vi "Main_07b.vi"() -> ()   [LabVIEW 2020]
uses:
  file_Item/MAP_Structure.ctl
  file_Item/Cluster_Item Data.ctl
  582f8871-3865-485f-b414-23c64cb36c00.vi
  acaf9b7b-e7cc-406a-a77a-e34bba61f78d.vi
  <vilib>/Comparison/Less/Less Functor/Less Functor.lvclass
  <vilib>/Comparison/Equal/Equal Functor/Equal Functor.lvclass
panel:
  out "index of element":i32
  out "\\ Size":u32
  out "sorted array":u32[](array[numeric])
  out "Selected dir size":u32
  out "target number for unused":u32
  out "Free Space":u32
  out "Map":T1
  out "array":string[](array[string])
  in  "Puzzle":string="$ cd /\n$ ls\n187585 dgflmqwt.srm\ndir gnpd\n200058 hbnlqs\ndir jsv\ndir mfhzl\ndir nljtr\ndir nwzp\n61949 qdswp.wfj\n21980 rbq.hpj\ndir rfwwwgr\ndir sbnhc\ndir zhfl\n136762 zwg\n$ cd gnpd\n$ ls\ndir dcqq\ndir dnscfz\ndir dwqbhgc\ndir lsrb\n167581 ndwfr.pbv\ndir pbgrdvmc\ndir sbnhc\n144703 sct\ndir smfhldss\n$ cd dcqq\n$ ls\ndir bfdng\n155230 mfhzl.bpw\ndir mhpqqq\ndir mpbpcv\n24140 mrrznmvr.mmz\n$ cd bfdng\n$ ls\ndir hjlch\ndir sbnhc\n$ cd hjlch\n$ ls\n239759 sct\n$ cd ..\n$ cd sbnhc\n$ ls\n221334 hbnlqs\n$ cd ..\n$ cd ..\n$ cd mhpqqq\n$ ls\n250305 nfqs.crt\ndir qqhz\n60892 rbq.hpj\n64587 tbzlnq\ndir tcbgmw\ndir vnlmlq\n$ cd qqhz\n$ ls\n148009 sct\n$ cd ..\n$ cd tcbgmw\n$ ls\n85006 sbnhc\n$ cd ..\n$ cd vnlmlq\n$ ls\n21720 vsrrhvlt.qbs\n$ cd ..\n$ cd ..\n$ cd mpbpcv\n$ ls\n146794 bdpld.ddm\n$ cd ..\n$ cd ..\n$ cd dnscfz\n$ ls\n276175 mfhzl.ndh\n248161 qjgzgm\ndir vnlmlq\ndir wwf\ndir zjdhldlq\n$ cd vnlmlq\n$ ls\n130051 ftjnfc\n$ cd ..\n$ cd wwf\n$ ls\n166550 dwvphbm.jtd\n$ cd ..\n$ cd zjdhldlq\n$ ls\n345090 hbnlqs\n$ cd ..\n$ cd ..\n$ cd dwqbhgc\n$ ls\n310228 dwvphbm\n157686 hbnlqs\n48014 nfqs.crt\n333356 rwb.njl\ndir sbnhc\n139174 sct\ndir vjcl\n$ cd sbnhc\n$ ls\n51605 bfqw.cjd\n267184 fjvmbpf\n169122 mfhzl.jrp\n243630 sbnhc\n$ cd ..\n$ cd vjcl\n$ ls\ndir mfhzl\n$ cd mfhzl\n$ ls\n302243 dcqq.djc\n$ cd ..\n$ cd ..\n$ cd ..\n$ cd lsrb\n$ ls\n311814 dcqq.prd\n200118 rbq.hpj\n$ cd ..\n$ cd pbgrdvmc\n$ ls\n119324 cqhdvmzp.npw\n277930 jhlrpmqg\ndir jlcqmq\n204425 pddmq\ndir rqmhwhc\n257084 sbnhc\n338348 vnlmlq\n$ cd jlcqmq\n$ ls\n24876 mfhzl\n$ cd ..\n$ cd rqmhwhc\n$ ls\n36575 dlft.dtp\n$ cd ..\n$ cd ..\n$ cd sbnhc\n$ ls\ndir sbq\ndir vmslnrmc\n$ cd sbq\n$ ls\n15689 hpzgsl.svb\n$ cd ..\n$ cd vmslnrmc\n$ ls\ndir lcqpws\n136481 nfqs.crt\n29838 sbnhc\n$ cd lcqpws\n$ ls\n168866 dcqq.pdp\n322264 jmtwr.fzj\n18732 sct\n$ cd ..\n$ cd ..\n$ cd ..\n$ cd smfhldss\n$ ls\ndir wfbssqj\n$ cd wfbssqj\n$ ls\n134050 tgghrp.hjq\n$ cd ..\n$ cd ..\n$ cd ..\n$ cd jsv\n$ ls\ndir bwc\ndir dcqq\n260913 lzcqm.wzr\ndir rhstw\ndir vnlmlq\n$ cd bwc\n$ ls\n221975 bdv.mfq\ndir crbnzrtw\ndir dcqq\ndir gdgh\n101246 gqcfrzmn\ndir gsst\ndir jwrhclh\ndir nbwfdvsv\ndir qnwhfv\ndir sbnhc\n$ cd crbnzrtw\n$ ls\ndir dmmpcrz\n204859 dwvphbm.csz\ndir jdh\ndir mpgdhg\n202360 nfqs.crt\ndir sbnhc\n302165 scpq.gpd\ndir shfhmdw\ndir wmjgmd\n$ cd dmmpcrz\n$ ls\ndir mfhzl\n$ cd mfhzl\n$ ls\n121861 hbnlqs\n$ cd ..\n$ cd ..\n$ cd jdh\n$ ls\ndir dwvphbm\n$ cd dwvphbm\n$ ls\n8977 ntdtdq\n$ cd ..\n$ cd ..\n$ cd mpgdhg\n$ ls\n48235 dcqq\n$ cd ..\n$ cd sbnhc\n$ ls\ndir dbb\n$ cd dbb\n$ ls\n275648 gcsdd.pdw\ndir rbbgrtm\ndir rmlm\n111336 sbnhc.qrn\n153146 sct\n$ cd rbbgrtm\n$ ls\n304685 rbq.hpj\n$ cd ..\n$ cd rmlm\n$ ls\ndir wfr\n$ cd wfr\n$ ls\n197220 dhjjr.dqq\n$ cd ..\n$ cd ..\n$ cd ..\n$ cd ..\n$ cd shfhmdw\n$ ls\n221308 mhnfzmz.gqp\n$ cd ..\n$ cd wmjgmd\n$ ls\ndir psrshrws\ndir zrtpgbg\n$ cd psrshrws\n$ ls\n202052 twgfblm\n$ cd ..\n$ cd zrtpgbg\n$ ls\n48134 hsnzvhvm.gnp\n$ cd ..\n$ cd ..\n$ cd ..\n$ cd dcqq\n$ ls\n63600 tlclsj.pvg\n181384 tzjn\n90096 wgq.lrm\n$ cd ..\n$ cd gdgh\n$ ls\n78450 hrcdgnpv.ctz\n$ cd ..\n$ cd gsst\n$ ls\n345240 nfqs.crt\n199259 sct\n$ cd ..\n$ cd jwrhclh\n$ ls\ndir ftjcr\n177499 nhdh.bbn\ndir sbnhc\ndir vnlmlq\ndir wqjnwgpj\n$ cd ftjcr\n$ ls\ndir glfptjpb\n121761 gqp\n36602 lcgfmtf.zct\ndir mfhzl\ndir rrrrgbqv\n236133 wdmwgzvs.jnw\ndir zwrmjlh\n$ cd glfptjpb\n$ ls\ndir fdnppcr\ndir gchhnd\ndir gdphvds\n98000 gqhv\n$ cd fdnppcr\n$ ls\ndir dwvphbm\ndir ngsgrgp\n$ cd dwvphbm\n$ ls\ndir wrg\n$ cd wrg\n$ ls\n265022 cqhdvmzp.npw\n316916 nfqs.crt\n$ cd ..\n$ cd ..\n$ cd ngsgrgp\n$ ls\n110198 sct\n$ cd ..\n$ cd ..\n$ cd gchhnd\n$ ls\n253836 hbnlqs\n39462 mfhzl\n211458 nfqs.crt\n$ cd ..\n$ cd gdphvds\n$ ls\ndir dpdb\n$ cd dpdb\n$ ls\n342610 vnlmlq\n$ cd ..\n$ cd ..\n$ cd ..\n$ cd mfhzl\n$ ls\ndir cptj\n$ cd cptj\n$ ls\n100729 nvctqj.gjw\n$ cd ..\n$ cd ..\n$ cd rrrrgbqv\n$ ls\n166055 dwvphbm.rvb\n303762 hbnlqs\n277411 wzr.rgz\n$ cd ..\n$ cd zwrmjlh\n$ ls\n32583 dvfnw\n$ cd ..\n$ cd ..\n$ cd sbnhc\n$ ls\ndir hwtmwp\n334229 mfhzl\n299303 vtrfbw.dng\n$ cd hwtmwp\n$ ls\ndir zjmrr\n$ cd zjmrr\n$ ls\n279103 cqhdvmzp.npw\n$ cd ..\n$ cd ..\n$ cd ..\n$ cd vnlmlq\n$ ls\ndir btqsh\ndir clhclcr\n237487 cqhdvmzp.npw\n11669 gqhltqf\n91205 hbnlqs\ndir qwbnvzv\n234450 rqlnhpc.qfd\ndir vbrc\ndir vfdqq\n$ cd btqsh\n$ ls\ndir lgh\ndir ljrjpg\n34333 rbq.hpj\n15387 vzldp.ffs\n$ cd lgh\n$ ls\n176966 vnlmlq\n$ cd ..\n$ cd ljrjpg\n$ ls\n231230 cqhdvmzp.npw\ndir dwvphbm\ndir mfhzl\n251554 rdrbn.clr\n180447 sbnhc\n$ cd dwvphbm\n$ ls\ndir vghvsmq\n$ cd vghvsmq\n$ ls\n132209 cqhdvmzp.npw\ndir jqmgn\n$ cd jqmgn\n$ ls\n95992 clbvg.bmr\n$ cd ..\n$ cd ..\n$ cd ..\n$ cd mfhzl\n$ ls\ndir dcqq\n$ cd dcqq\n$ ls\ndir vjhl\n$ cd vjhl\n$ ls\ndir nbhmzl\n$ cd nbhmzl\n$ ls\n155454 sbnhc.flh\n$ cd ..\n$ cd ..\n$ cd ..\n$ cd ..\n$ cd ..\n$ cd ..\n$ cd clhclcr\n$ ls\ndir jwqwhq\n268077 njcmcfl.ctm\n$ cd jwqwhq\n$ ls\n256988 rbq.hpj\n$ cd ..\n$ cd ..\n$ cd qwbnvzv\n$ ls\n167852 dln.zrn\ndir hpwpm\n131149 lsc.tjj\ndir mfhzl\ndir mzhwwrtp\n201277 sbnhc.pfh\n147232 zlmgttpl\n$ cd hpwpm\n$ ls\n135194 jpzt.fjn\n$ cd ..\n$ cd mfhzl\n$ ls\n166015 jrcqvgf.jdg\n$ cd ..\n$ cd mzhwwrtp\n$ ls\n231983 dgrvfdmp\n121846 dwvphbm.lvp\n$ cd ..\n$ cd ..\n$ cd vbrc\n$ ls\n320029 wbhs.mpd\n$ cd ..\n$ cd vfdqq\n$ ls\n277998 nfqs.crt\ndir qzgwglhc\ndir vnlmlq\n68520 wsc.vhz\ndir zfdhthfn\n$ cd qzgwglhc\n$ ls\n25046 cqhdvmzp.npw\n250876 dwvphbm\n$ cd ..\n$ cd vnlmlq\n$ ls\n212688 hbnlqs\n8202 mlpl.tsp\n69495 vnlmlq.thv\n281200 vzdwr.tbl\n$ cd ..\n$ cd zfdhthfn\n$ ls\n233242 dstb.hrs\n269387 nfqs.crt\n$ cd ..\n$ cd ..\n$ cd ..\n$ cd wqjnwgpj\n$ ls\ndir hfd\ndir lbft\ndir rtlw\ndir vbf\n$ cd hfd\n$ ls\n224694 cqhdvmzp.npw\n100103 dbmwn.tqz\n$ cd ..\n$ cd lbft\n$ ls\n60107 hbnlqs\n$ cd ..\n$ cd rtlw\n$ ls\ndir ntpb\n$ cd ntpb\n$ ls\n341166 mfhzl.pvj\n$ cd ..\n$ cd ..\n$ cd vbf\n$ ls\n54177 ghrscj.tlh\n$ cd ..\n$ cd ..\n$ cd ..\n$ cd nbwfdvsv\n$ ls\n107273 mptw.qmn\n$ cd ..\n$ cd qnwhfv\n$ ls\n55633 hbnlqs\n$ cd ..\n$ cd sbnhc\n$ ls\n173163 vnlmlq\n$ cd ..\n$ cd ..\n$ cd dcqq\n$ ls\n217679 hbnlqs\n146747 ltp\n$ cd ..\n$ cd rhstw\n$ ls\ndir clh\ndir grz\ndir ntjtzr\ndir qrjgl\ndir rzqp\ndir tzgrs\ndir zrdh\n$ cd clh\n$ ls\n212153 cqhdvmzp.npw\n$ cd ..\n$ cd grz\n$ ls\n346002 cqhdvmzp.npw\n$ cd ..\n$ cd ntjtzr\n$ ls\n271549 rbq.hpj\n308693 sbnhc.zrv\n$ cd ..\n$ cd qrjgl\n$ ls\n119344 jfshwj\n$ cd ..\n$ cd rzqp\n$ ls\n327891 dcqq\n210282 hlmnv.jph\n118199 nfqs.crt\ndir rwh\n$ cd rwh\n$ ls\n285057 rmvrnb\n$ cd ..\n$ cd ..\n$ cd tzgrs\n$ ls\n23830 cjqrr\n$ cd ..\n$ cd zrdh\n$ ls\ndir dcqq\ndir dwvphbm\n188911 rbq.hpj\ndir vpnzs\n$ cd dcqq\n$ ls\n277454 hbnlqs\ndir jnncgzgm\n$ cd jnncgzgm\n$ ls\n199664 dcqq.tgm\n$ cd ..\n$ cd ..\n$ cd dwvphbm\n$ ls\n221700 fgnznr.dhf\n$ cd ..\n$ cd vpnzs\n$ ls\n254459 fvcf.zcj\n$ cd ..\n$ cd ..\n$ cd ..\n$ cd vnlmlq\n$ ls\ndir gfsj\n$ cd gfsj\n$ ls\ndir hddvr\n$ cd hddvr\n$ ls\ndir mqmnzb\n$ cd mqmnzb\n$ ls\n341835 jjjh\n$ cd ..\n$ cd ..\n$ cd ..\n$ cd ..\n$ cd ..\n$ cd mfhzl\n$ ls\ndir pccldwf\n$ cd pccldwf\n$ ls\n126977 nvcw\n318605 rljpfnc.dzd\n$ cd ..\n$ cd ..\n$ cd nljtr\n$ ls\ndir slztzqd\n$ cd slztzqd\n$ ls\n55754 bpwghjpg.bfq\n205753 pfplh\n319151 vdlmjj.mmn\ndir vnlmlq\n$ cd vnlmlq\n$ ls\ndir mfhzl\n338081 zhjrrs\ndir zpj\n$ cd mfhzl\n$ ls\ndir dcqq\ndir lgfb\ndir rjbprpnl\n343125 vnlmlq.zpr\n$ cd dcqq\n$ ls\n288030 rbq.hpj\n$ cd ..\n$ cd lgfb\n$ ls\n22119 cqhdvmzp.npw\n238775 wbmnzgt.vnl\n$ cd ..\n$ cd rjbprpnl\n$ ls\n244896 lvgg.jvz\n$ cd ..\n$ cd ..\n$ cd zpj\n$ ls\n339679 dcqq\n$ cd ..\n$ cd ..\n$ cd ..\n$ cd ..\n$ cd nwzp\n$ ls\ndir mfhzl\ndir vnlmlq\n$ cd mfhzl\n$ ls\n107297 dwvphbm.nvb\n$ cd ..\n$ cd vnlmlq\n$ ls\ndir mdj\n$ cd mdj\n$ ls\n87553 dbtct.nws\n$ cd ..\n$ cd ..\n$ cd ..\n$ cd rfwwwgr\n$ ls\n287719 flpwrp\n74896 mfhzl\n$ cd ..\n$ cd sbnhc\n$ ls\n232949 dcqq.rnj\ndir dwvphbm\n$ cd dwvphbm\n$ ls\n21955 pcqbfbv.bfg\n$ cd ..\n$ cd ..\n$ cd zhfl\n$ ls\ndir jvnlhq\ndir vnlmlq\n180619 wcd.jsr\n$ cd jvnlhq\n$ ls\n20692 clp.vmd\ndir dbn\n91389 jqbp.zss\ndir njmdrb\ndir sbnhc\ndir sdrrzp\n192374 vnlmlq.lvj\n$ cd dbn\n$ ls\n293401 dcqq\n$ cd ..\n$ cd njmdrb\n$ ls\n270463 dvzbtnbb.vth\ndir gdvtg\n219739 hsdg.rss\ndir mfhzl\n285584 mhq\ndir mllvdccz\n234503 nfqs.crt\n$ cd gdvtg\n$ ls\n294243 dllnh\n27407 rws.vqt\n$ cd ..\n$ cd mfhzl\n$ ls\ndir dwvphbm\n154477 nbphv.pjc\ndir qpnncj\n33994 splscqn.tqz\ndir vnlmlq\n$ cd dwvphbm\n$ ls\n87960 sct\n$ cd ..\n$ cd qpnncj\n$ ls\n182692 lqbbz\n$ cd ..\n$ cd vnlmlq\n$ ls\n285614 bfrjhpv.dvn\n121146 nfqs.crt\n84544 sbnhc\n$ cd ..\n$ cd ..\n$ cd mllvdccz\n$ ls\n184878 bsjzsmw.pwt\n184061 dcqq.bbm\n243546 dwvphbm.rdw\ndir ftmrszgl\n8251 rbq.hpj\ndir tgvchzn\n$ cd ftmrszgl\n$ ls\n267439 bdrn.gfb\n257447 npcrg.gjn\n$ cd ..\n$ cd tgvchzn\n$ ls\n227775 lqbftlg.scr\n$ cd ..\n$ cd ..\n$ cd ..\n$ cd sbnhc\n$ ls\n245520 tjp.pml\n$ cd ..\n$ cd sdrrzp\n$ ls\ndir dcqq\n7894 gstzs\ndir rnjcrjj\ndir sbnhc\n$ cd dcqq\n$ ls\n340987 sjb.nss\n$ cd ..\n$ cd rnjcrjj\n$ ls\n67782 rbq.hpj\n$ cd ..\n$ cd sbnhc\n$ ls\n156705 zwr.rtg\n$ cd ..\n$ cd ..\n$ cd ..\n$ cd vnlmlq\n$ ls\ndir dwvphbm\ndir jgc\ndir lbh\ndir lrwt\ndir rhszw\n213882 sbnhc.dzl\ndir vnlmlq\n2798 vwwbhsnb.dms\n$ cd dwvphbm\n$ ls\n257972 zccsn.bdr\n$ cd ..\n$ cd jgc\n$ ls\n85911 cqhdvmzp.npw\ndir fnvjv\n49760 grsw\ndir ntz\n249818 rgzqq.tlr\n$ cd fnvjv\n$ ls\n288935 dcqq.bsq\ndir nwlbbwtq\n264238 tcwwzs.zwg\n$ cd nwlbbwtq\n$ ls\ndir qcm\n318151 sbnhc.lwr\n322077 stb.cqj\n$ cd qcm\n$ ls\n147721 crrdn\ndir gctnt\n59476 rbq.hpj\ndir sbnhc\n$ cd gctnt\n$ ls\n328909 dwvphbm\n82536 rjnz\n$ cd ..\n$ cd sbnhc\n$ ls\n35956 nfqs.crt\n89464 qvhvlcl.nzq\ndir vvn\n$ cd vvn\n$ ls\n119247 fztlb.qch\n79030 vnlmlq\n$ cd ..\n$ cd ..\n$ cd ..\n$ cd ..\n$ cd ..\n$ cd ntz\n$ ls\n234879 mfhzl\n$ cd ..\n$ cd ..\n$ cd lbh\n$ ls\ndir dwvphbm\n24310 jgsp.ggs\ndir lft\n$ cd dwvphbm\n$ ls\n295434 rbq.hpj\n$ cd ..\n$ cd lft\n$ ls\ndir dcqq\ndir dwvphbm\n123657 mfhzl.nhq\n$ cd dcqq\n$ ls\ndir tgp\n$ cd tgp\n$ ls\n271647 gmmq.tmp\n$ cd ..\n$ cd ..\n$ cd dwvphbm\n$ ls\ndir pftcdtd\n108321 qtqhqwnt\n$ cd pftcdtd\n$ ls\n28073 hwqzcr.zcp\n$ cd ..\n$ cd ..\n$ cd ..\n$ cd ..\n$ cd lrwt\n$ ls\n38953 hzhzfw.tpv\n59885 vnlmlq\n$ cd ..\n$ cd rhszw\n$ ls\ndir hsfbh\ndir mmflqvsd\n20071 rhdbms\n162563 rpjjld\ndir vnlmlq\n$ cd hsfbh\n$ ls\n255050 lglw.jvw\n99814 pzvw\n28443 sbct.hng\n168934 sbnhc.fnt\ndir wnwztl\n$ cd wnwztl\n$ ls\ndir brwhjj\n215806 dcqq\n214967 mqhv.wwq\n82998 vcm.mhc\n$ cd brwhjj\n$ ls\n171935 rbq.hpj\n$ cd ..\n$ cd ..\n$ cd ..\n$ cd mmflqvsd\n$ ls\n109141 dcqq.mdc\n$ cd ..\n$ cd vnlmlq\n$ ls\ndir blggqt\n117656 dcqq.vlg\ndir fpw\n195879 gsb.dvw\ndir mfhzl\n5068 mnfdf\ndir mtg\ndir vnlmlq\n$ cd blggqt\n$ ls\n195700 ntv.zjn\n$ cd ..\n$ cd fpw\n$ ls\n143105 sct\n$ cd ..\n$ cd mfhzl\n$ ls\ndir cpcczt\n47767 nzzcn.qhp\ndir zdv\n$ cd cpcczt\n$ ls\n209755 vnlmlq.lbw\n$ cd ..\n$ cd zdv\n$ ls\n335546 sbnhc.ccg\n$ cd ..\n$ cd ..\n$ cd mtg\n$ ls\n244632 dcqq.frr\n240873 tpvqthc.ljw\ndir zdtnqtcw\n$ cd zdtnqtcw\n$ ls\n80980 nfqs.crt\n$ cd ..\n$ cd ..\n$ cd vnlmlq\n$ ls\n153953 dwvphbm\n$ cd ..\n$ cd ..\n$ cd ..\n$ cd vnlmlq\n$ ls\ndir dcqq\ndir dwvphbm\n155333 mmhjscr.mrh\n293720 nfqs.crt\ndir qnv\ndir rdvq\n226720 zgmtqvws\n160920 zgnft\n$ cd dcqq\n$ ls\n142227 cqhdvmzp.npw\n199798 twqppvs\n$ cd ..\n$ cd dwvphbm\n$ ls\n58807 cdbdnrqh.fgq\n224321 hbnlqs\n340073 sbnhc\n337932 sct\n2613 vdc.nwz\n$ cd ..\n$ cd qnv\n$ ls\n244311 cqhdvmzp.npw\n273687 jhqt.glz\ndir mnrh\n240044 nfqs.crt\n49861 pwsgmlq.hcw\ndir rdrs\n126195 vnlmlq.frr\n$ cd mnrh\n$ ls\n276125 hbnlqs\n$ cd ..\n$ cd rdrs\n$ ls\ndir dqgw\n213018 dwvphbm\n13785 hbnlqs\ndir lbpjczw\n116081 nfqs.crt\n154367 rbq.hpj\n77634 sct\n$ cd dqgw\n$ ls\ndir rpcfdr\n$ cd rpcfdr\n$ ls\ndir swvlhbg\n$ cd swvlhbg\n$ ls\n309244 sct\n$ cd ..\n$ cd ..\n$ cd ..\n$ cd lbpjczw\n$ ls\n69436 rbq.hpj\n$ cd ..\n$ cd ..\n$ cd ..\n$ cd rdvq\n$ ls\n128806 dcqq.qzr\n64132 dcqq.vgc\ndir hht\n165359 jzj.rqv\ndir sbnhc\n$ cd hht\n$ ls\ndir vnlmlq\n$ cd vnlmlq\n$ ls\n49895 wct\n$ cd ..\n$ cd ..\n$ cd sbnhc\n$ ls\n265434 vnlmlq"
  in  "Example":string="$ cd /\n$ ls\ndir a\n14848514 b.txt\n8504156 c.dat\ndir d\n$ cd a\n$ ls\ndir e\n29116 f\n2557 g\n62596 h.lst\n$ cd e\n$ ls\n584 i\n$ cd ..\n$ cd ..\n$ cd d\n$ ls\n4060174 j\n8033020 d.log\n5626152 d.ext\n7214296 k"
  # "10475598."
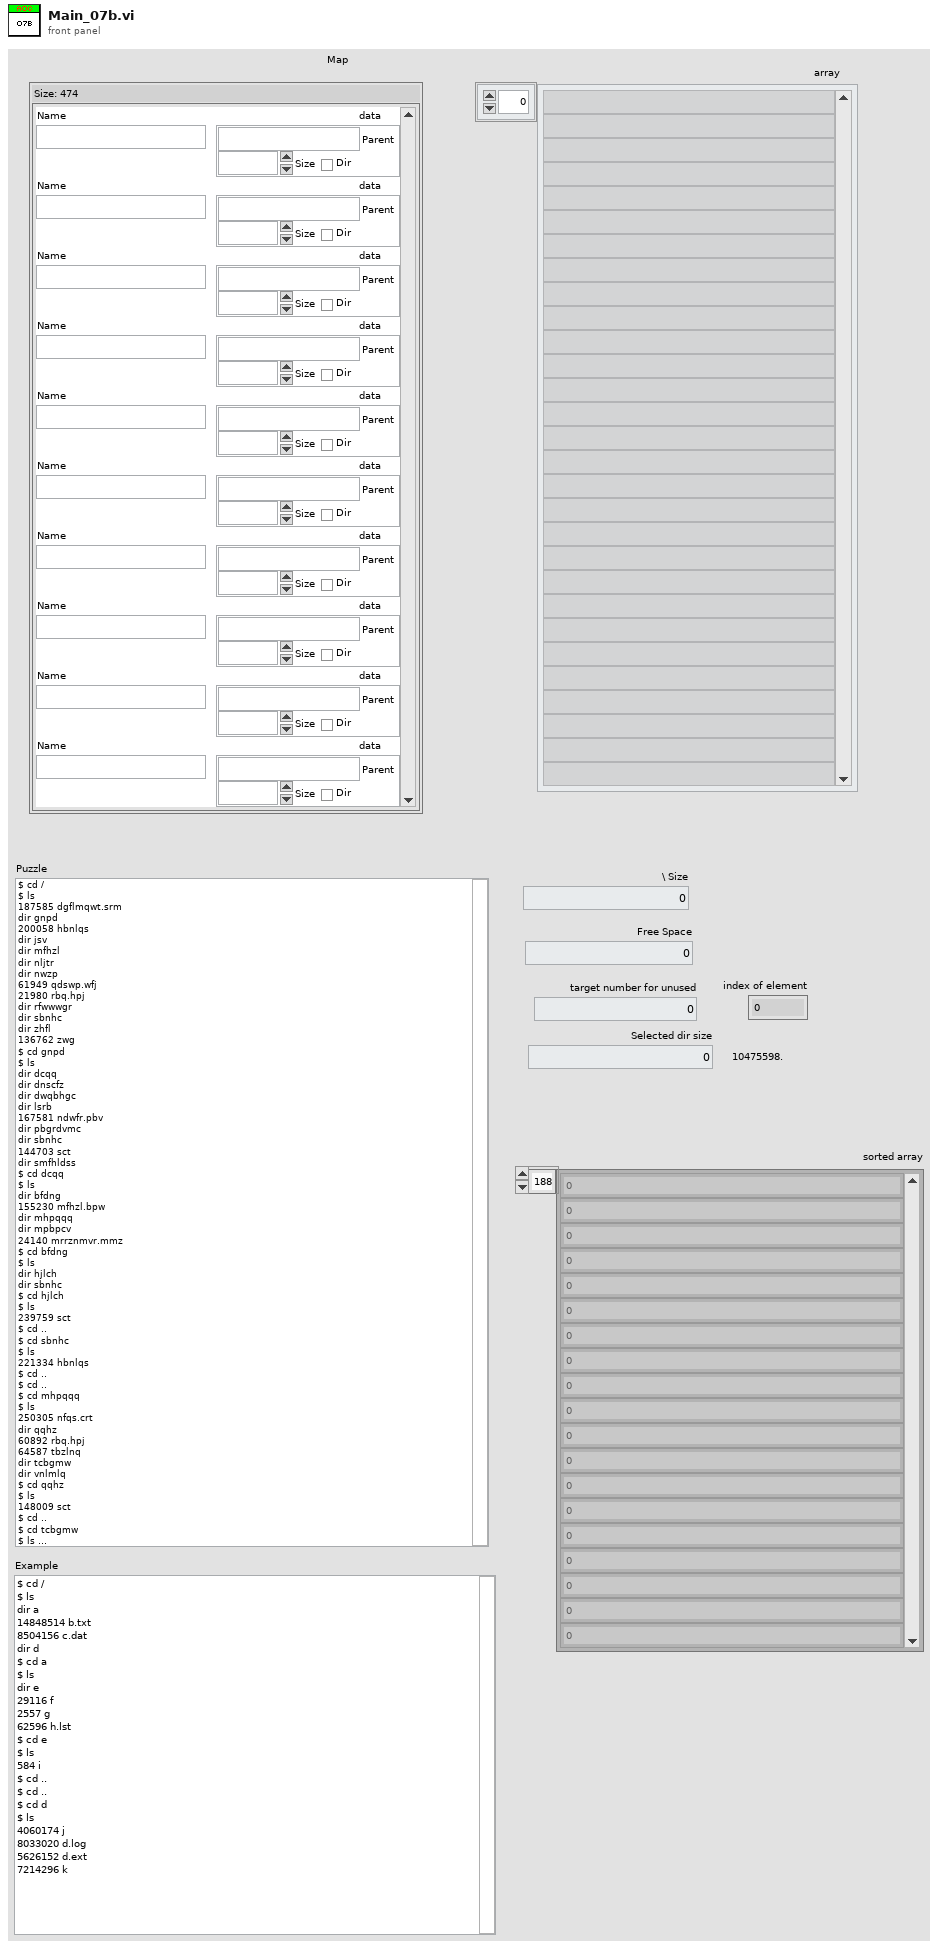
[diagram p1: front panel]
types:
  T1 = typedef "MAP_Structure.ctl" = map{string, T2}
  T2 = typedef "Cluster_Item Data.ctl" = cluster{"Parent":string, "Size":u32, "Dir":bool}
  T3 = cluster{"Parent":string, "Item Array":cluster{"Dir":bool, "Name":string, "Size":i32}[]}
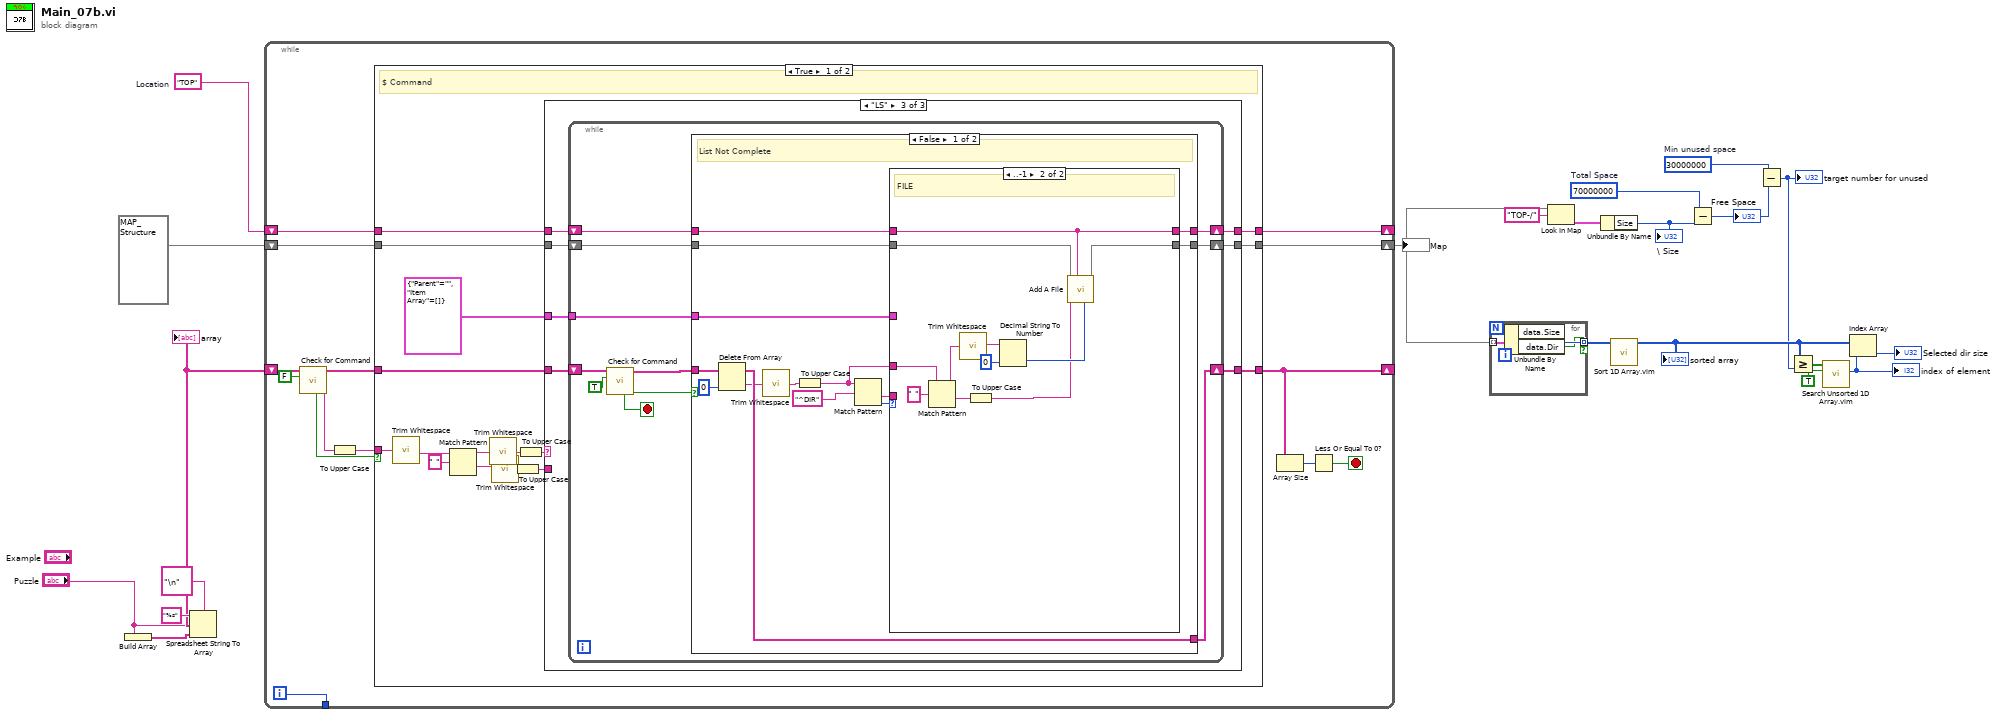
[diagram p0: block diagram]
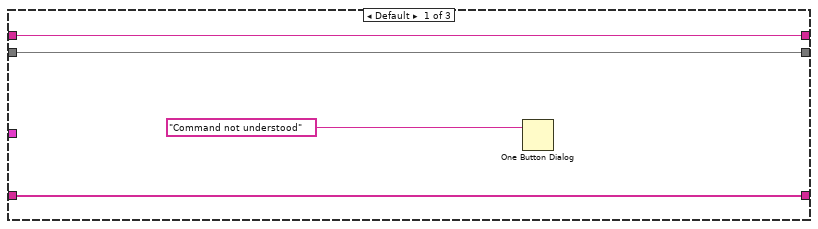
[diagram p2: hidden frame]
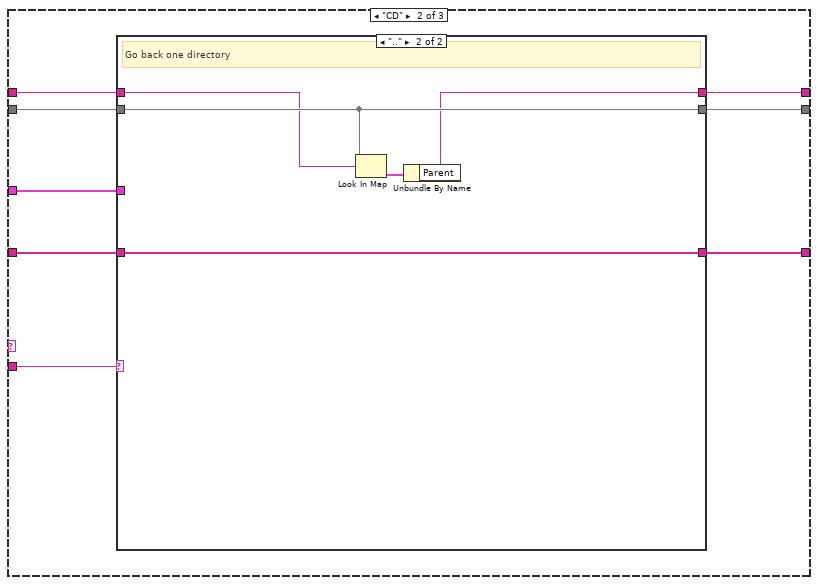
[diagram p3: hidden frame]
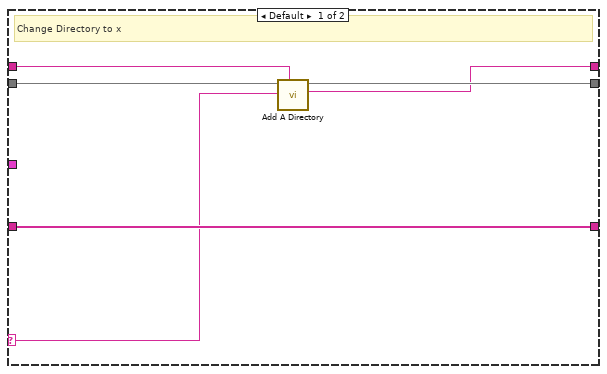
[diagram p4: hidden frame]
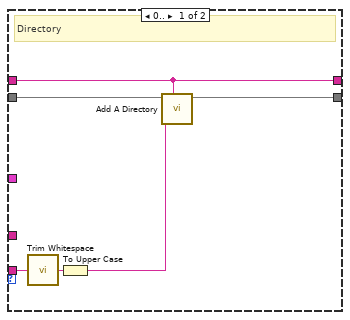
[diagram p5: hidden frame]
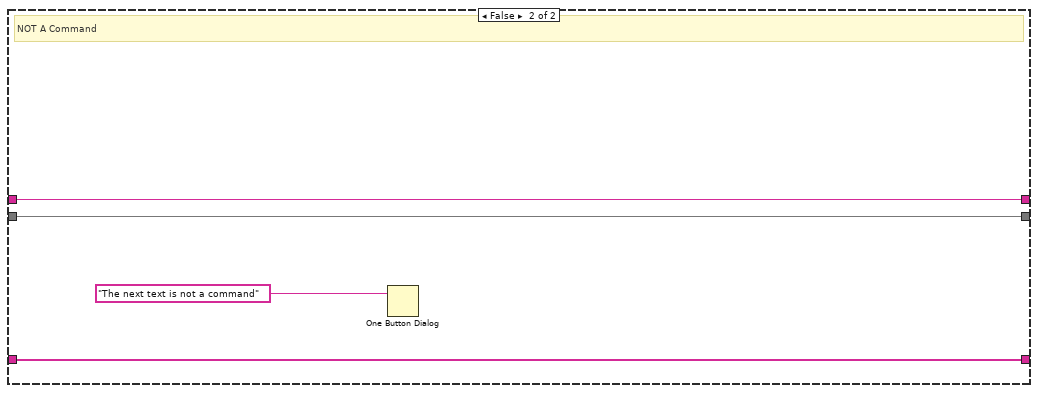
[diagram p7: hidden frame]
diagram:
  w13 = u32 70000000  # Total Space
  w11 = u32 30000000  # Min unused space
  w17 = "TOP"  # Location
  n1 = Build Array("Puzzle") -> (w21:string[])
  n2 = Spreadsheet String To Array(delimiter (Tab)="\n", format string="%s", spreadsheet string="Puzzle", array type (2D Dbl)=w21) -> (array=w16:string[])
  "array" <- w16
  n3 = while {
    shift-right: [w26] -> _
    shift-left: w16 -> [w31]
    shift-right: [w34] -> w10
    shift-left: T1 {} -> [w35]
    shift-right: [w32] -> _
    shift-left: w17 -> [w33]
    tunnel: [w22] -> _
    i -> [w22]
    stop <- w24 stop-if-true
    n4 = call "Check for Command.vi"("Check Only"=FALSE, "Array"=w31) -> ("Argument Out"=w29:string, "Array Out"=w30:string[], "Found Out"=w28:bool)  [unwired: 7 in]
    n5 = To Upper Case(1:w29) -> (0:w23:string)
    n6 = case shown="True" w28 {
      tunnel: w30 -> [w43 w128]
      tunnel: w35 -> [w41 w129]
      tunnel: [w40 w129] -> w34
      tunnel: [w42 w128] -> w26
      tunnel: w23 -> [w51 _]
      tunnel: w33 -> [w39 w126]
      tunnel: [w38 w126] -> w32
      frame True {
        # "$ Command"
        n7 = call <vilib>:"Trim Whitespace.vi"("string"=w51) -> ("trimmed string"=w50:string)  [unwired: 1 in]
        n8 = Match Pattern(string=w50, regular expression=" ") -> (before substring=w48:string, after substring=w46:string)  [unwired: 1 in, 2 out]
        n9 = call <vilib>:"Trim Whitespace.vi"("string"=w48) -> ("trimmed string"=w47:string)  [unwired: 1 in]
        n10 = call <vilib>:"Trim Whitespace.vi"("string"=w46) -> ("trimmed string"=w45:string)  [unwired: 1 in]
        n11 = To Upper Case(1:w45) -> (0:w36:string)
        n12 = To Upper Case(1:w47) -> (0:w44:string)
        n13 = case shown="\"LS\"" w44 {
          tunnel: w36 -> [_ w61 _]
          tunnel: w43 -> [w55 w60 w77]
          tunnel: [w55 w59 w76] -> w42
          tunnel: w41 -> [w54 w62 w81]
          tunnel: [w54 w63 w78] -> w40
          tunnel: w39 -> [w52 w58 w80]
          tunnel: [w52 w57 w79] -> w38
          tunnel: T3 {"Parent"="", "Item Array"=[]} ("value") -> [_ w56 w75]
          frame Default {
            n14 = One Button Dialog(message="Command not understood") -> ()  [unwired: 1 in, 1 out]
          }
          frame "CD" {
            n15 = case shown="\"..\"" w61 {
              selector: w61 -> [w65 _]
              tunnel: [w68 w73] -> w63
              tunnel: w62 -> [w67 w73]
              tunnel: w60 -> [w69 w74]
              tunnel: [w69 w74] -> w59
              tunnel: w58 -> [w66 w70]
              tunnel: [w64 w71] -> w57
              tunnel: w56 -> [_ _]
              frame Default {
                # "Change Directory to x"
                n16 = call "Add A Directory.vi"("Parrent"=w66, "Name"=w65, "Map"=w67) -> ("Dir Name Out"=w64:string, "Map Out"=w68:T1)  [unwired: 7 in]
              }
              frame ".." {
                # "Go back one directory"
                n17 = Look In Map(map=w73, key=w70) -> (value=w72:T2)  [unwired: 1 in, 1 out]
                n18 = Unbundle By Name(w72) -> ("Parent"=w71:string)
              }
            }
          }
          frame "LS" {
            n19 = while {
              shift-right: [w83] -> w78
              shift-left: w81 -> [w88]
              shift-right: [w84] -> w79
              shift-left: w80 -> [w89]
              shift-right: [w86] -> w76
              shift-left: w77 -> [w91]
              tunnel: w75 -> [w85]
              stop <- w82 stop-if-true
              n20 = call "Check for Command.vi"("Check Only"=TRUE, "Array"=w91) -> ("Array Out"=w87:string[], "Found Out"=w82:bool)  [unwired: 7 in, 1 out]
              n21 = case shown="False" w82 {
                tunnel: w89 -> [w98 w123]
                tunnel: w88 -> [w97 w124]
                tunnel: w87 -> [w105 w125]
                tunnel: [w103 w125] -> w86
                tunnel: w85 -> [w94 _]
                tunnel: [w93 w123] -> w84
                tunnel: [w92 w124] -> w83
                frame False {
                  # "List Not Complete"
                  n22 = Delete From Array(array=w105, index=0) -> (deleted portion=w102:string, array with subset deleted=w103:string[])  [unwired: 1 in]
                  n23 = call <vilib>:"Trim Whitespace.vi"("string"=w102) -> ("trimmed string"=w101:string)  [unwired: 1 in]
                  n24 = To Upper Case(1:w101) -> (0:w95:string)
                  n25 = Match Pattern(string=w95, regular expression="^DIR") -> (after substring=w96:string, offset past match=w99:i32)  [unwired: 1 in, 2 out]
                  n26 = case shown="..-1" w99 {
                    tunnel: w98 -> [w110 w114]
                    tunnel: w97 -> [w111 w120]
                    tunnel: w96 -> [w109 _]
                    tunnel: w95 -> [_ w122]
                    tunnel: w94 -> [_ _]
                    tunnel: [w110 w114] -> w93
                    tunnel: [w107 w119] -> w92
                    frame 0.. {
                      # "Directory"
                      n27 = call <vilib>:"Trim Whitespace.vi"("string"=w109) -> ("trimmed string"=w108:string)  [unwired: 1 in]
                      n28 = To Upper Case(1:w108) -> (0:w106:string)
                      n29 = call "Add A Directory.vi"("Parrent"=w110, "Name"=w106, "Map"=w111) -> ("Map Out"=w107:T1)  [unwired: 7 in, 1 out]
                    }
                    frame ..-1 {
                      # "FILE"
                      n30 = Match Pattern(string=w122, regular expression=" ") -> (before substring=w118:string, after substring=w113:string)  [unwired: 1 in, 2 out]
                      n31 = call <vilib>:"Trim Whitespace.vi"("string"=w118) -> ("trimmed string"=w117:string)  [unwired: 1 in]
                      n32 = To Upper Case(1:w113) -> (0:w112:string)
                      n33 = Decimal String To Number(string=w117, default (0L)=u32 0 ("default (0 I32)")) -> (number=w115:u32)  [unwired: 1 in, 1 out]
                      n34 = call "Add A File.vi"("Size"=w115, "Parrent"=w114, "Name"=w112, "Map"=w120) -> ("Map Out"=w119:T1)  [unwired: 7 in]
                    }
                  }
                }
                frame True {
                  # "List Complete"
                }
              }
            }
          }
        }
      }
      frame False {
        # "NOT A Command"
        n35 = One Button Dialog(message="The next text is not a command") -> ()  [unwired: 1 in, 1 out]
      }
    }
    n36 = Array Size(array=w26) -> (size(s)=w25:i32)
    n37 = Less Or Equal To 0?(x=w25) -> (x <= 0?=w24:bool)
  }
  "Map" <- w10
  n38 = for {
    tunnel: w10 -> [w132] mode=indexing
    tunnel: [w131] -> w9 mode=indexing if=w130
    n39 = Unbundle By Name(w132) -> ("data.Size"=w131:u32, "data.Dir"=w130:bool)
  }
  n40 = Look In Map(map=w10, key="TOP-/") -> (value=w14:T2)  [unwired: 1 in, 1 out]
  n41 = Unbundle By Name(w14) -> ("Size"=w12:u32)
  "\\ Size" <- w12
  n42 = call "Sort 1D Array.vim"("unsorted array"=w9) -> ("sorted array"=w5:u32[])  [unwired: 10 in]
  "sorted array" <- w5
  n43 = Subtract(x=w13, y=w12) -> (x-y=w3:u32)
  "Free Space" <- w3
  n44 = Subtract(x=w11, y=w3) -> (x-y=w1:u32)
  "target number for unused" <- w1
  n45 = Greater Or Equal?(x=w5, y=w1) -> (x >= y?=w8:bool[])
  n46 = call "Search Unsorted 1D Array.vim"("element"=TRUE, "unsorted 1D array"=w8) -> ("index of element"=w6:i32)  [unwired: 9 in]
  "index of element" <- w6
  n47 = Index Array(array=w5, index=w6) -> (element=→"Selected dir size":u32)
